vi "writeDBL.vi"(8 "error in (no error)":errorcluster, 10 "Input":dbl, 11 "ModbusBuffer in":refnum<class "ModbusBuffer.lvclass">) -> (0 "error out":errorcluster, 3 "ModbusBuffer out":refnum<class "ModbusBuffer.lvclass">)   [LabVIEW 2016, in "RTModbus.lvlib" / "ModbusBuffer.lvclass"]
uses:
  ModbusBuffer.lvclass
  ModbusBuffer.lvclass/ModbusBuffer.ctl
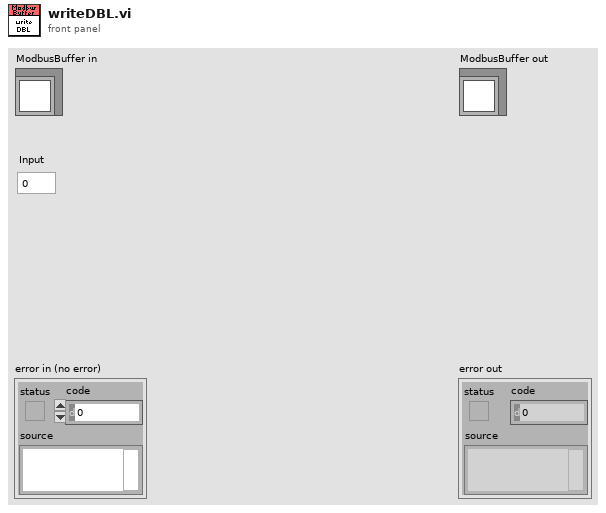
[diagram p1: front panel]
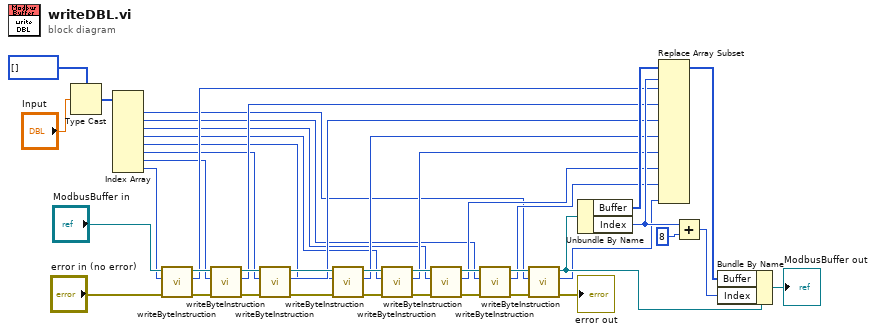
[diagram p0: block diagram]
diagram:
  n1 = Type Cast(type=u8[] [], x="Input") -> (*(type *) &x=w9:u8[])
  n2 = Index Array(array=w9) -> (element #1=w8:u8, element #2=w7:u8, element #3=w6:u8, element #4=w5:u8, element #5=w4:u8, element #6=w3:u8, element #7=w2:u8, element #8=w1:u8)  [unwired: 8 in]
  n3 = call "writeByteInstruction.vi"("error in (no error)"="error in (no error)", "Input"=w1, "ModbusBuffer in"="ModbusBuffer in") -> ("error out"=w25:errorcluster, "Output"=w12:u16, "ModbusBuffer out"=w36:refnum<class "ModbusBuffer.lvclass">)  [unwired: 6 in]
  n4 = call "writeByteInstruction.vi"("error in (no error)"=w25, "Input"=w2, "ModbusBuffer in"=w36) -> ("error out"=w24:errorcluster, "Output"=w13:u16, "ModbusBuffer out"=w35:refnum<class "ModbusBuffer.lvclass">)  [unwired: 6 in]
  n5 = call "writeByteInstruction.vi"("error in (no error)"=w24, "Input"=w3, "ModbusBuffer in"=w35) -> ("error out"=w23:errorcluster, "Output"=w14:u16, "ModbusBuffer out"=w34:refnum<class "ModbusBuffer.lvclass">)  [unwired: 6 in]
  n6 = call "writeByteInstruction.vi"("error in (no error)"=w23, "Input"=w4, "ModbusBuffer in"=w34) -> ("error out"=w22:errorcluster, "Output"=w15:u16, "ModbusBuffer out"=w33:refnum<class "ModbusBuffer.lvclass">)  [unwired: 6 in]
  n7 = call "writeByteInstruction.vi"("error in (no error)"=w22, "Input"=w5, "ModbusBuffer in"=w33) -> ("error out"=w21:errorcluster, "Output"=w16:u16, "ModbusBuffer out"=w32:refnum<class "ModbusBuffer.lvclass">)  [unwired: 6 in]
  n8 = call "writeByteInstruction.vi"("error in (no error)"=w21, "Input"=w6, "ModbusBuffer in"=w32) -> ("error out"=w20:errorcluster, "Output"=w17:u16, "ModbusBuffer out"=w31:refnum<class "ModbusBuffer.lvclass">)  [unwired: 6 in]
  n9 = call "writeByteInstruction.vi"("error in (no error)"=w20, "Input"=w7, "ModbusBuffer in"=w31) -> ("error out"=w19:errorcluster, "Output"=w28:u16, "ModbusBuffer out"=w30:refnum<class "ModbusBuffer.lvclass">)  [unwired: 6 in]
  n10 = call "writeByteInstruction.vi"("error in (no error)"=w19, "Input"=w8, "ModbusBuffer in"=w30) -> ("error out"=→"error out":errorcluster, "Output"=w27:u16, "ModbusBuffer out"=w29:refnum<class "ModbusBuffer.lvclass">)  [unwired: 6 in]
  n11 = Unbundle By Name(w29) -> ("Buffer"=w41:u16[], "Index"=w39:i32)
  n12 = Replace Array Subset(array=w41, new element #1=w12, index #1=w39, new element #2=w13, new element #3=w14, new element #4=w15, new element #5=w16, new element #6=w17, new element #7=w28, new element #8=w27) -> (w40:u16[])  [unwired: 7 in]
  n13 = Add(x=w39, y=8) -> (x+y=w42:i32)
  n14 = Bundle By Name(cluster=w29, "Buffer"=w40, "Index"=w42) -> (→"ModbusBuffer out":refnum<class "ModbusBuffer.lvclass">)
